vi "执行校准.vi"(3 "校准点位":u16(ring) caption="校准方式：" items=["第一点校准", "第二点校准", "第三点校准"], 5 "校准方式":u16(ring) caption="校准方式：" items=["单点校准", "两点校准", "三点校准"], 6 "校准量程":u16, 7 "校准参数":u16(ring) caption="校准参数：" items=["pH", "DO", "浊度", "电导率", "叶绿素a", "藻密度", "ORP", "DO2"], 8 "error in (no error)":errorcluster caption="错误输入（无错误）", 9 "标液三":cluster{"标准值":dbl, "检测值":dbl, "原始值":dbl} caption="标液三：" {"原始值" format="%#.6f"; "检测值" format="%#.6f"; "标准值" format="%#.6f"}, 10 "标液二":cluster{"标准值":dbl, "检测值":dbl, "原始值":dbl} caption="标液二：" {"原始值" format="%#.6f"; "检测值" format="%#.6f"; "标准值" format="%#.6f"}, 11 "标液一":cluster{"标准值":dbl, "检测值":dbl, "原始值":dbl} caption="标液一：" {"原始值" format="%#.6f"; "检测值" format="%#.6f"; "标准值" format="%#.6f"}) -> (0 "error out":errorcluster)   [LabVIEW 2016, in "斯坦道多参数.lvlib"]
panel:
  in  "选项卡控件":enum32{"选项卡 1"}(tab)
  # "检测值"
  # "原始值"
  # "标准值"
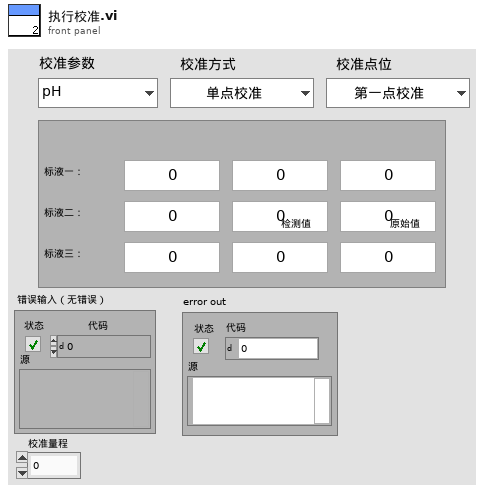
[diagram p1: front panel]
types:
  T1 = cluster{"pH探头选择":u16, "DO探头选择":u16, "电导率探头选择":u16, "浊度探头选择":u16, "叶绿素a探头选择":u16, "蓝绿藻探头选择":u16, "orp探头选择":u16, "COD探头选择":u16, "DO2探头选择":u16}
  T2 = enum16{"NULL", "pH", "Cond", "DO", "Turb", "ORP"}
  T3 = enum16{"null", "pH", "DO", "浊度", "电导率", "叶绿素a", "藻密度"}
  T4 = enum16{"null", "pH", "DO", "浊度", "电导率", "叶绿素a", "DO2"}
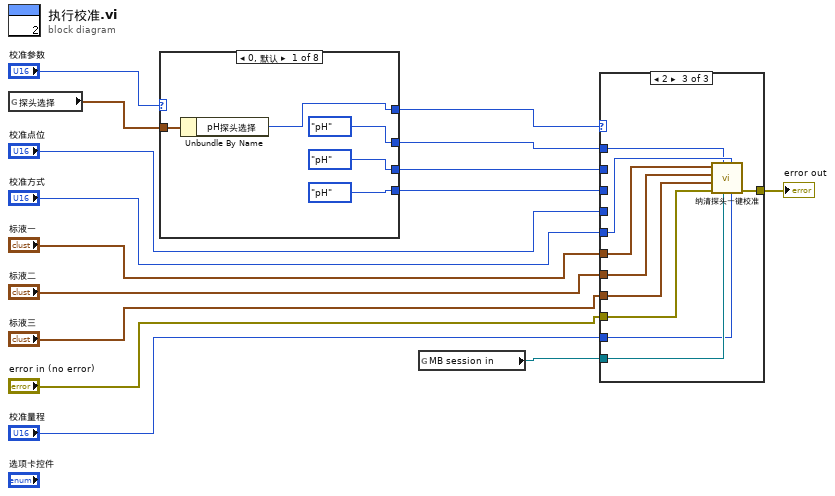
[diagram p0: block diagram]
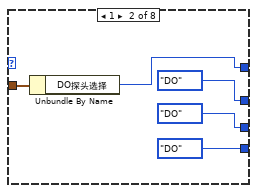
[diagram p2: hidden frame]
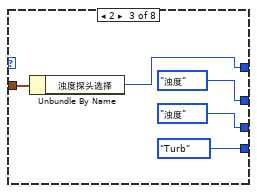
[diagram p3: hidden frame]
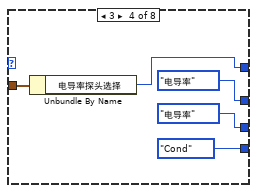
[diagram p4: hidden frame]
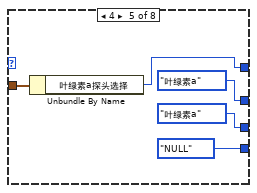
[diagram p5: hidden frame]
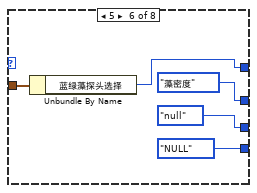
[diagram p6: hidden frame]
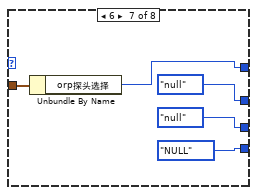
[diagram p7: hidden frame]
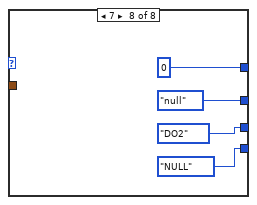
[diagram p8: hidden frame]
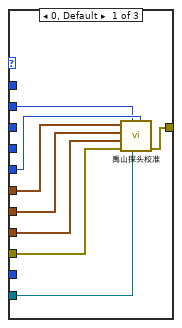
[diagram p9: hidden frame]
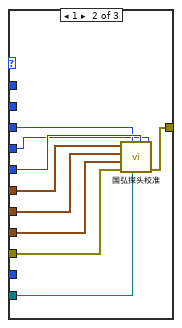
[diagram p10: hidden frame]
diagram:
  n1 = global read "断电保存变量.vi" "探头选择"() -> (w6:T1)
  n2 = case shown="0, 默认" "校准参数" {
    tunnel: [T4."pH" ("探头") T4."DO" ("探头") T4."浊度" ("探头") T4."电导率" ("探头") T4."叶绿素a" ("探头") T4."null" ("探头") T4."null" ("探头") T4."DO2" ("探头")] -> w7
    tunnel: w6 -> [w19 w24 w29 w34 w40 w44 w49 _]
    tunnel: [w18 w23 w28 w33 w39 w43 w48 u16 0 ("orp探头选择")] -> w5
    tunnel: [T3."pH" ("探头") T3."DO" ("探头") T3."浊度" ("探头") T3."电导率" ("探头") T3."叶绿素a" ("探头") T3."藻密度" ("探头") T3."null" ("探头") T3."null" ("探头")] -> w4
    tunnel: [T2."pH" ("探头") T2."DO" ("探头") T2."Turb" ("探头") T2."Cond" ("探头") T2."NULL" ("探头") T2."NULL" ("探头") T2."NULL" ("探头") T2."NULL" ("探头")] -> w3
    frame 0, Default {
      n3 = Unbundle By Name(w19) -> ("pH探头选择"=w18:u16)
    }
    frame 1 {
      n4 = Unbundle By Name(w24) -> ("DO探头选择"=w23:u16)
    }
    frame 2 {
      n5 = Unbundle By Name(w29) -> ("浊度探头选择"=w28:u16)
    }
    frame 3 {
      n6 = Unbundle By Name(w34) -> ("电导率探头选择"=w33:u16)
    }
    frame 4 {
      n7 = Unbundle By Name(w40) -> ("叶绿素a探头选择"=w39:u16)
    }
    frame 5 {
      n8 = Unbundle By Name(w44) -> ("蓝绿藻探头选择"=w43:u16)
    }
    frame 6 {
      n9 = Unbundle By Name(w49) -> ("orp探头选择"=w48:u16)
    }
    frame 7 {
    }
  }
  n10 = global read "多参数全局变量.vi" "MB session in"() -> (w15:refnum<class "MB_Master.lvclass">)
  n11 = case shown="2" w5 {
    tunnel: w15 -> [w56 w69 w74]
    tunnel: [w62 w70 w80] -> w14
    tunnel: "标液一" -> [w57 w67 w78]
    tunnel: "error in (no error)" -> [w61 w71 w79]
    tunnel: "标液二" -> [w60 w66 w77]
    tunnel: "标液三" -> [w59 w65 w76]
    tunnel: "校准方式" -> [w58 w68 w75]
    tunnel: w7 -> [w55 _ _]
    tunnel: w4 -> [_ _ w73]
    tunnel: w3 -> [_ w64 _]
    tunnel: "校准点位" -> [_ w63 _]
    tunnel: "校准量程" -> [_ _ w72]
    frame 0, Default {
      n12 = call "禹山探头校准.vi"("校准方式"=w58, "MB_Master输入"=w56, "探头"=w55, "错误输入（无错误）"=w61, "标液三"=w59, "标液二"=w60, "标液一"=w57) -> ("错误输出"=w62:errorcluster)  [unwired: 4 in]
    }
    frame 1 {
      n13 = call "国弘探头校准.vi"("校准点位"=w63, "校准方式"=w68, "MB_Master输入"=w69, "探头"=w64, "错误输入（无错误）"=w71, "标液三"=w65, "标液二"=w66, "标液一"=w67) -> ("错误输出"=w70:errorcluster)  [unwired: 3 in]
    }
    frame 2 {
      n14 = call "纳清探头一键校准.vi"("校准量程"=w72, "校准方式"=w75, "MB_Master输入"=w74, "探头"=w73, "error in (no error)"=w79, "标液三"=w76, "标液二"=w77, "标液一"=w78) -> ("error out"=w80:errorcluster)  [unwired: 3 in]
    }
  }
  "error out" <- w14
